vi "validate configuration.vi"(8 "error in":errorcluster, 11 "Scan Engine configuration in":refnum<class "Scan Engine configuration.lvclass">) -> (0 "error out":errorcluster, 3 "Scan Engine configuration out":refnum<class "Scan Engine configuration.lvclass">)   [LabVIEW 2013, in "Scan Engine configuration.lvclass"]
doc: "This function performs validation of the configuration. This function should be safe to call at any point and should not rely on anything in the runtime environment."
uses:
  Scan Engine configuration.lvclass
  <vilib>/NI/Tag Bus Module Framework/module configuration/TBM module configuration.lvclass
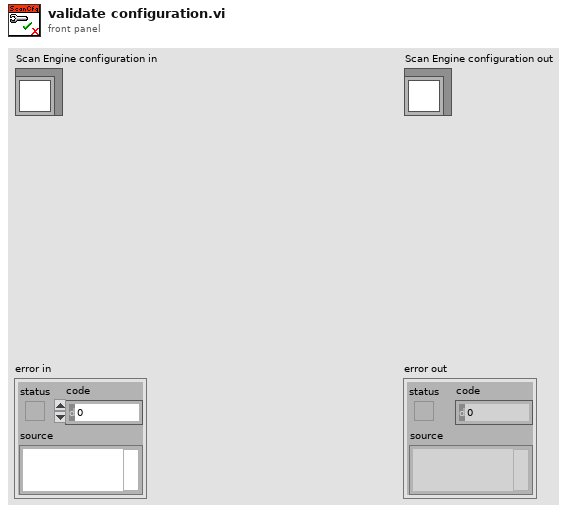
[diagram p1: front panel]
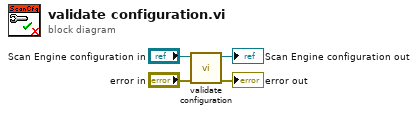
[diagram p0: block diagram]
diagram:
  n1 = call-parent "validate configuration.vi"("error in"="error in", "configuration in"="Scan Engine configuration in") -> ("error out"=→"error out":errorcluster, "configuration out"=→"Scan Engine configuration out":refnum<class "Scan Engine configuration.lvclass">)  [unwired: 8 in]
